vi "Scale Data.vi"(8 "error in (no error)":errorcluster, 10 "Data":T1, 11 "Data Processor Module in":refnum<class "Data Processor Module.lvclass">) -> (0 "error out":errorcluster, 2 "Scaled Data":T1, 3 "Data Processor Module out":refnum<class "Data Processor Module.lvclass">)   [LabVIEW 2020, in "VolatusData.lvlib" / "Data Processor Module.lvclass"]
uses:
  Data Processor Module.lvclass
  Data Processor Module.lvclass/Data Processor Module.ctl
  Scaling/Scaling.lvclass
  New Data.ctl
  VolatusData.lvlib
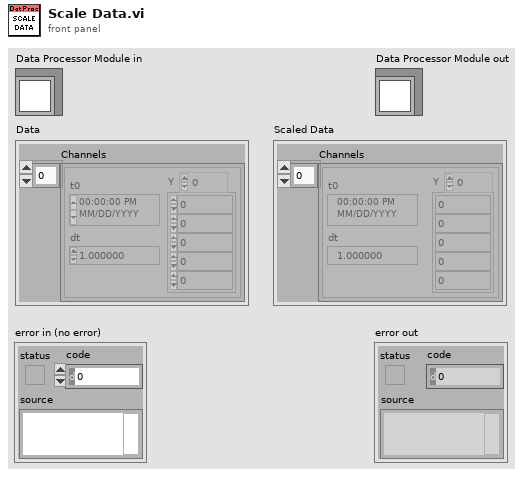
[diagram p1: front panel]
types:
  T1 = typedef "VolatusData.lvlib/New Data.ctl" = cluster{"Channels":waveform(dbl)[]}
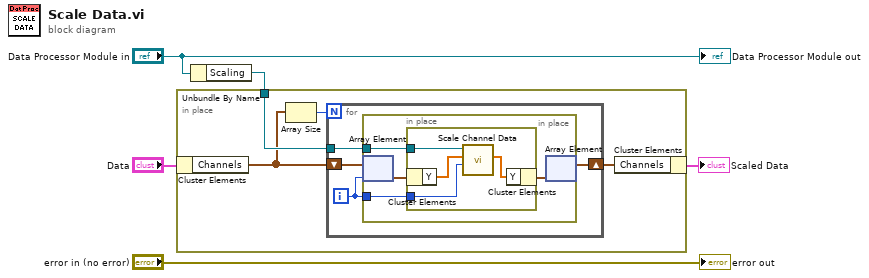
[diagram p0: block diagram]
diagram:
  n1 = Unbundle By Name("Data Processor Module in") -> ("Scaling"=w3:refnum<class "Scaling.lvclass">)
  n2 = in-place {
    in-place-border: w3 -> [w9]
    n3 = in-place-cluster #1("Data") -> ("Channels"=w7:waveform(dbl)[])
    n4 = Array Size(array=w7) -> (size(s)=w6:i32)
    n5 = for {
      N: w6 -> [_]
      tunnel: w9 -> [w13]
      shift-right: [w10] -> w8
      shift-left: w7 -> [w12]
      i -> [w11]
      n6 = in-place {
        in-place-border: w13 -> [w17]
        in-place-border: w11 -> [w15]
        n7 = in-place-array #2(w12, w11) -> (w16:waveform(dbl))
        n8 = in-place {
          in-place-border: w17 -> [w21]
          in-place-border: w15 -> [w19]
          n9 = in-place-cluster #3(w16) -> ("Y"=w20:dbl[])
          n10 = call "Scale Channel Data.vi"("Channel Index"=w19, "Data"=w20, "Scaling in"=w21) -> ("Scaled Data"=w18:dbl[])  [unwired: 6 in, 2 out]
          n11 = in-place-cluster #3("Y"=w18) -> (w14:waveform(dbl))
        }
        n12 = in-place-array #2(w14) -> (w10:waveform(dbl)[])  [unwired: 1 out]
      }
    }
    n13 = in-place-cluster #1("Channels"=w8) -> (→"Scaled Data":T1)
  }
  "error out" <- "error in (no error)"
  "Data Processor Module out" <- "Data Processor Module in"
